vi "Configure Ethernet.vi"(8 "Error In":errorcluster, 10 "TCP Configuration":T1={"IP Address"="10.2.106.227", "Port"=927}, 11 "LINX Device Config":T2) -> (0 "Error Out":errorcluster, 3 "LINX Device Config":T2)   [LabVIEW 2020, in "Device.lvlib"]
doc: "Configure the LINX device's Ethernet settings."
uses:
  Device.lvlib
  Type Defs/Interface.ctl
  LMH-LINX.lvlib
  Type Defs/Channels.ctl
  Type Defs/TCP Config.ctl
  Type Defs/LINX Device Config.ctl
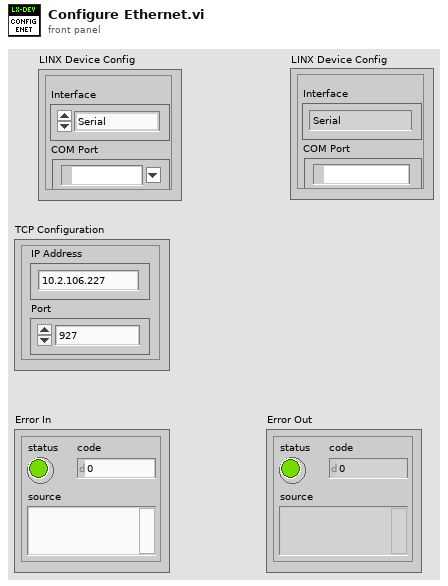
[diagram p1: front panel]
types:
  T1 = typedef "Device.lvlib/TCP Config.ctl" = cluster{"IP Address":string, "Port":u16}
  T2 = typedef "Device.lvlib/LINX Device Config.ctl" = cluster{"Interface":T3, "COM Port":refnum<visa-resource-name>, "TCP Configuration":T1, "Device Family":u8, "Device ID":u8, "Device Name":string, "TCP Ref":refnum<k5>, "Channels":T4}
  T3 = typedef "LMH-LINX.lvlib/Interface.ctl" = enum16{"Serial", "TCP"}
  T4 = typedef "LMH-LINX.lvlib/Channels.ctl" = cluster{"DI":u8[], "DO":u8[], "AI":u8[], "AO":u8[], "PWM":u8[], "QE":u8[], "UART":u8[], "I2C 2":u8[], "SPI":u8[], "CAN":u8[], "Servo":u8[], "AI Ref (V)":dbl, "AI Resolution (Bits)":u8, "AO Ref (V)":dbl, "AO Resolution (Bits)":u8}
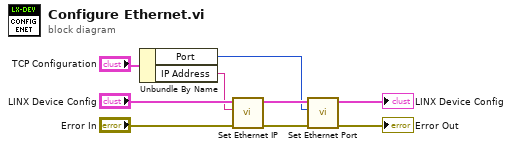
[diagram p0: block diagram]
diagram:
  n1 = Unbundle By Name("TCP Configuration") -> ("Port"=w2:u16, "IP Address"=w1:string)
  n2 = call "Set Ethernet IP.vi"("Error In"="Error In", "IP Address"=w1, "LINX Device Config"="LINX Device Config") -> ("Error Out"=w8:errorcluster, "LINX Device Config"=w9:T2)  [unwired: 7 in]
  n3 = call "Set Ethernet Port.vi"("Error In"=w8, "Port"=w2, "LINX Device Config"=w9) -> ("Error Out"=→"Error Out":errorcluster, "LINX Device Config"=→"LINX Device Config":T2)  [unwired: 7 in]
